vi "Wait.vi"(8 "error in (no error)":errorcluster, 9 "Timeout (-1ms)":i32=-1, 11 "Response Core in":refnum<class "Response Core.lvclass">) -> (0 "error out":errorcluster, 1 "Timeout?":bool, 3 "Response Core out":refnum<class "Response Core.lvclass">)   [LabVIEW 2020, in "Publisher.lvlib" / "Response Core.lvclass"]
doc: "Execute a wait on the Response Core. \n\nThe default implementation uses a standard wait function and is not interruptible."
uses:
  Response Core.lvclass
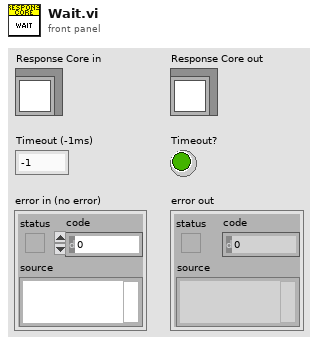
[diagram p1: front panel]
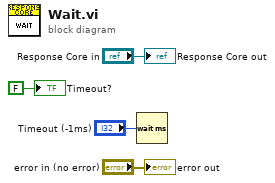
[diagram p0: block diagram]
diagram:
  n1 = Wait (ms)(milliseconds to wait="Timeout (-1ms)") -> ()  [unwired: 1 out]
  "error out" <- "error in (no error)"
  "Response Core out" <- "Response Core in"
  "Timeout?" <- FALSE ("Dropped?")
